vi "SubVI-AOMvolt-Power Calibration for 1064-noglobal.vi"(0 "Min voltage (V)":dbl=0.5, 1 "instrument handle":refnum<visa-resource-name>, 2 "Max voltage (V)":dbl=4.5, 3 "scan step #":dbl=25.0, 4 "error in (no error)":errorcluster {"code" format="%.0x"}, 5 "milliseconds to wait":u32=200) -> (6 "output cluster":T1, 7 "Polynomial Coefficients":dbl[](array[numeric]) format="%0.2f")   [LabVIEW 2014]
uses:
  <vilib>/Utility/file.llb/Write To Spreadsheet File (DBL).vi
  <vilib>/Analysis/NI_AALPro.lvlib
panel:
  out "Cal-Power (mW)":dbl[](array[numeric])
  out "Cal-AOM (V)":dbl[](array[numeric])
  out "Power-AOM Graph":T2(graph)
  out "Voltage to AOM (V)":dbl
  out "Power readout (mW)":dbl
  out "Scan size per step (V)":dbl=0.25
  in  "save cal curve?":bool
  # "**activate \ncontinuous power\ncontinuous AOM"
  # "continuous scaning power \nover AOM voltage range"
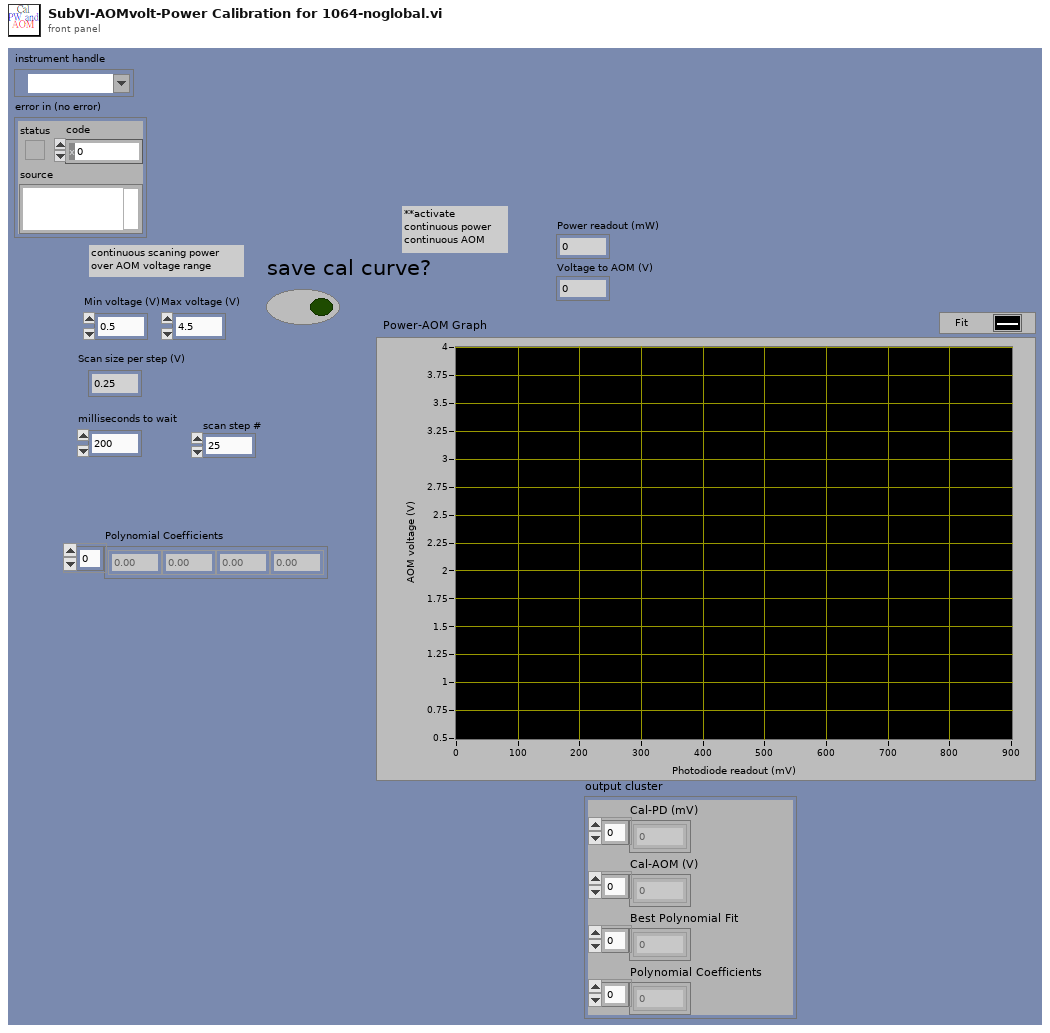
[diagram p1: front panel]
types:
  T1 = cluster{"Cal-PD (mV)":dbl[], "Cal-AOM (V)":dbl[], "Best Polynomial Fit":dbl[], "Polynomial Coefficients":dbl[]}
  T2 = cluster{"Cal-PD (mV)":dbl[], "Cal-AOM (V)":dbl[]}[]
  T3 = cluster{"Cal-Power (mW)":dbl[], "Best Polynomial Fit":dbl[]}
  T4 = cluster{"Cal-Power (mW)":dbl[], "Cal-AOM (V)":dbl[]}
  T5 = cluster{"Cal-Power (mW)":dbl[], "Cal-AOM (V)":dbl[], "Best Polynomial Fit":dbl[], "Polynomial Coefficients":dbl[]}
  T6 = cluster{"Cal-Power (mW)":dbl[], "Cal-AOM (V)":dbl[]}[]
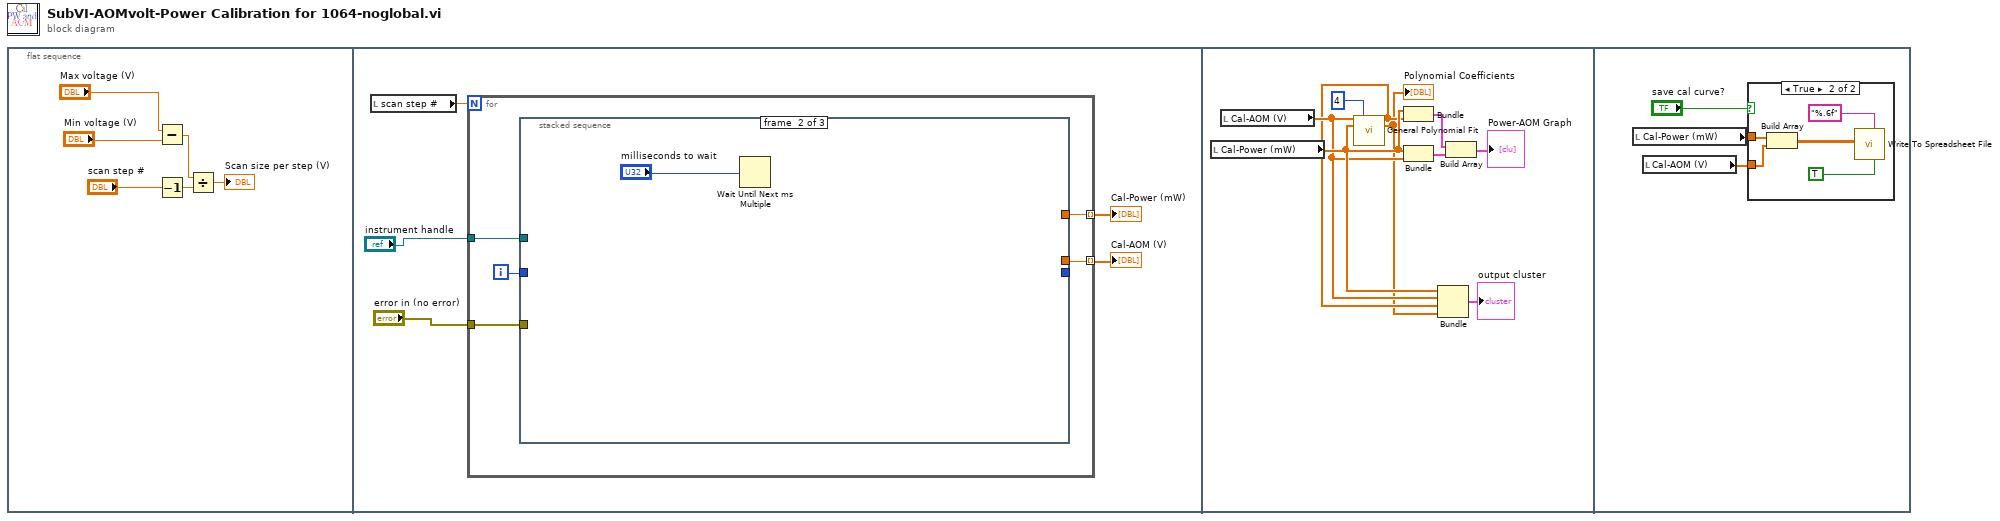
[diagram p0: block diagram]
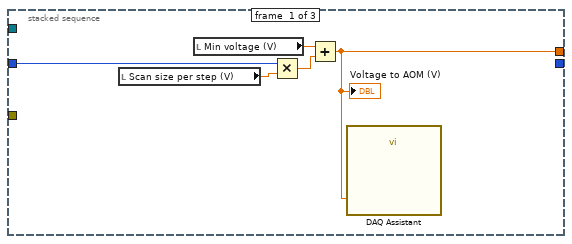
[diagram p2: hidden frame]
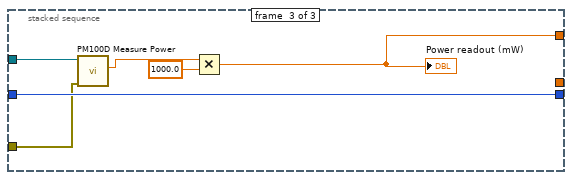
[diagram p3: hidden frame]
diagram:
  n1 = flat-sequence {
    frame #0 {
      n2 = Subtract(x="Max voltage (V)", y="Min voltage (V)") -> (x-y=w3:dbl)
      n3 = Decrement(x="scan step #") -> (x-1=w5:dbl)
      n4 = Divide(x=w3, y=w5) -> (x/y=→"Scan size per step (V)":dbl)
    }
    frame #1 {
      n5 = local read "scan step #"() -> (w11:dbl)
      n6 = for {
        N: w11 -> [_]
        tunnel: [w15] -> w9 mode=indexing
        tunnel: [w14] -> w10 mode=indexing
        tunnel: "instrument handle" -> [w13]
        tunnel: "error in (no error)" -> [w12]
        i -> [w16]
        n7 = stacked-sequence {
          tunnel: w16 -> [w18 _ w28]
          tunnel: [_ _ w28] -> _
          tunnel: [_ _ w23] -> w15
          tunnel: [w21 _ _] -> w14
          tunnel: w13 -> [_ _ w27]
          tunnel: w12 -> [_ _ w26]
          frame #0 {
            n8 = local read "Scan size per step (V)"() -> (w19:dbl)
            n9 = local read "Min voltage (V)"() -> (w20:dbl)
            n10 = Multiply(x=w18, y=w19) -> (x*y=w17:dbl)
            n11 = Add(x=w20, y=w17) -> (x+y=w21:dbl)
            "Voltage to AOM (V)" <- w21
            n12 = call "DAQ Assistant"("data"=w21) -> ()  [unwired: 17 in, 2 out]
          }
          frame #1 {
            n13 = Wait Until Next ms Multiple(millisecond multiple="milliseconds to wait") -> ()  [unwired: 1 out]
          }
          frame #2 {
            n14 = call <instrlib>:"PM100D Measure Power.vi"("error in (no error)"=w26, "instrument handle"=w27) -> ("Power"=w25:dbl)  [unwired: 7 in, 2 out]
            n15 = Multiply(x=w25, y=1000.0) -> (x*y=w23:dbl)
            "Power readout (mW)" <- w23
          }
        }
      }
      "Cal-AOM (V)" <- w10
      "Cal-Power (mW)" <- w9
    }
    frame #2 {
      n16 = local read "Cal-Power (mW)"() -> (w33:dbl[])
      n17 = local read "Cal-AOM (V)"() -> (w32:dbl[])
      n18 = call <vilib>:"General Polynomial Fit.vi"("Y"=w32, "polynomial order"=4, "X"=w33) -> ("Best Polynomial Fit"=w31:dbl[], "Polynomial Coefficients"=w30:dbl[])  [unwired: 9 in, 2 out]
      "Polynomial Coefficients" <- w30
      n19 = Bundle("Cal-Power (mW)"=w33, "Best Polynomial Fit"=w31) -> (w36:T3)  [unwired: 1 in]
      n20 = Bundle("Cal-Power (mW)"=w33, "Cal-AOM (V)"=w32) -> (w35:T4)  [unwired: 1 in]
      n21 = Bundle("Cal-Power (mW)"=w33, "Cal-AOM (V)"=w32, "Best Polynomial Fit"=w31, "Polynomial Coefficients"=w30) -> (→"output cluster":T5)  [unwired: 1 in]
      n22 = Build Array(w36, w35) -> (→"Power-AOM Graph":T6)
    }
    frame #3 {
      n23 = local read "Cal-Power (mW)"() -> (w39:dbl[])
      n24 = local read "Cal-AOM (V)"() -> (w38:dbl[])
      n25 = case shown="True" "save cal curve?" {
        tunnel: w39 -> [_ w44]
        tunnel: w38 -> [_ w43]
        frame False {
        }
        frame True {
          n26 = Build Array(w44, w43) -> (w42:dbl[][])
          n27 = call-poly <vilib>:"Write To Spreadsheet File.vi"("transpose? (no:F)"=TRUE, "format (%.3f)"="%.6f", "2D data"=w42) -> ()  [unwired: 3 in, 3 out]
        }
      }
    }
  }
